vi "3458 4ohm.vi"(1 "NRDGS":i32, 2 "error in (no error)":errorcluster, 3 "NPLC":u16(ring)=2 items=["10", "20", "50", "100", "200"], 4 "Multímetro TRP":string="22") -> (0 "error out":errorcluster)   [LabVIEW 2014]
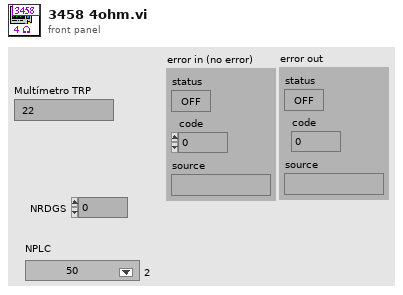
[diagram p1: front panel]
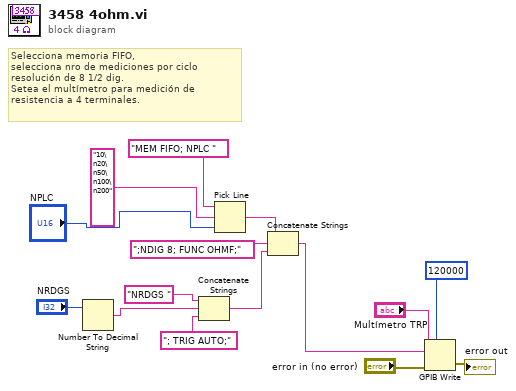
[diagram p0: block diagram]
diagram:
  # "Selecciona memoria FIFO,                         selecciona nro de mediciones por ciclo       resolución de 8 1/2 dig.                                 Setea el multímetro para medición de resistencia a 4 terminales."
  n1 = Number To Decimal String(number="NRDGS") -> (decimal integer string=w3:string)  [unwired: 1 in]
  n2 = Concatenate Strings("NRDGS ", w3, "; TRIG AUTO;") -> (w2:string)
  n3 = Pick Line(string ("")="MEM FIFO; NPLC " ("write buffer (\"\")"), multi-line string="10\n20\n50\n100\n200", line index="NPLC") -> (output string=w11:string)
  n4 = Concatenate Strings(w11, ";NDIG 8; FUNC OHMF;" ("Substring"), w2) -> (w7:string)
  n5 = GPIB Write(0:"Multímetro TRP", 1:w7, 3:"error in (no error)", 4:120000 ("timeout ms (488.2 global)")) -> (6:→"error out":errorcluster)  [unwired: 1 in, 1 out]
